vi "Set Measurement Rate.vi"(8 "error in (no error)":errorcluster, 9 "Measurement Rate (Hz)":u8(ring) items=["1 Hz", "5 Hz", "10 Hz"], 11 "Honeywell Compass HMC6343":refnum<class "Honeywell Compass HMC6343.lvclass">) -> (0 "error out":errorcluster, 3 "Honeywell Compass HMC6343 out":refnum<class "Honeywell Compass HMC6343.lvclass">)   [LabVIEW 2019, in "Honeywell Compass HMC6343.lvclass"]
doc: "Changes the Run Mode Measurement Rate of the device. There are three options : 1Hz, 5Hz, 10Hz. The factory value is 5Hz."
uses:
  Honeywell Compass HMC6343.lvclass
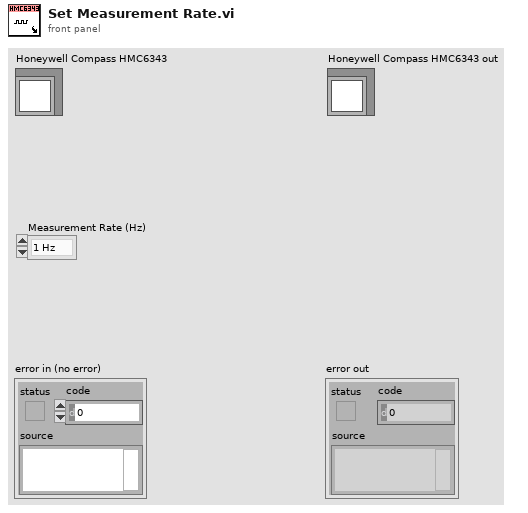
[diagram p1: front panel]
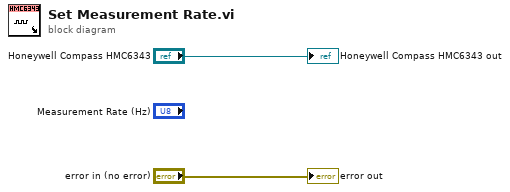
[diagram p0: block diagram]
diagram:
  "error out" <- "error in (no error)"
  "Honeywell Compass HMC6343 out" <- "Honeywell Compass HMC6343"
